vi "Lambda NOx.vi"(10 "O2 meas":dbl) -> (2 "Lambda":dbl)   [LabVIEW 2011]
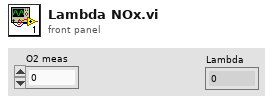
[diagram p1: front panel]
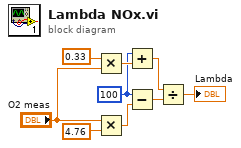
[diagram p0: block diagram]
diagram:
  w4 = 100
  n1 = Multiply(x=0.33, y="O2 meas") -> (x*y=w8:dbl)
  n2 = Multiply(x="O2 meas", y=4.76) -> (x*y=w5:dbl)
  n3 = Add(x=w4, y=w8) -> (x+y=w3:dbl)
  n4 = Subtract(x=w4, y=w5) -> (x-y=w2:dbl)
  n5 = Divide(x=w3, y=w2) -> (x/y=→"Lambda":dbl)
